vi "Enable-Disable.vi"(8 "error in (no error)":errorcluster, 10 "State":enum16{"Init", "Account Verified"}(ring), 11 "Control/Indicator References":T1) -> (0 "error out":errorcluster)   [LabVIEW 2020]
doc: "This VI enables/disables controls and indicators."
uses:
  Controls/Controls-Indicators References.ctl
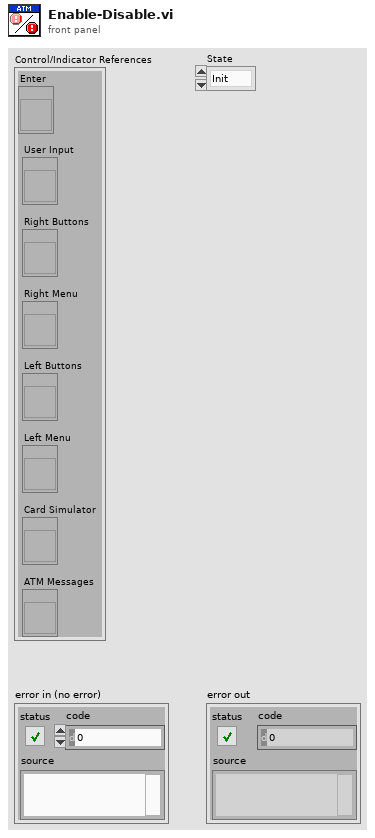
[diagram p1: front panel]
types:
  T1 = typedef "Controls-Indicators References.ctl" = cluster{"Enter":refnum<vi>, "User Input":refnum<vi>, "Right Buttons":refnum<vi>, "Right Menu":refnum<vi>, "Left Buttons":refnum<vi>, "Left Menu":refnum<vi>, "Card Simulator":refnum<vi>, "ATM Messages":refnum<vi>}
  T2 = enum8{"Enabled", "Disabled", "Disabled and Grayed Out"}
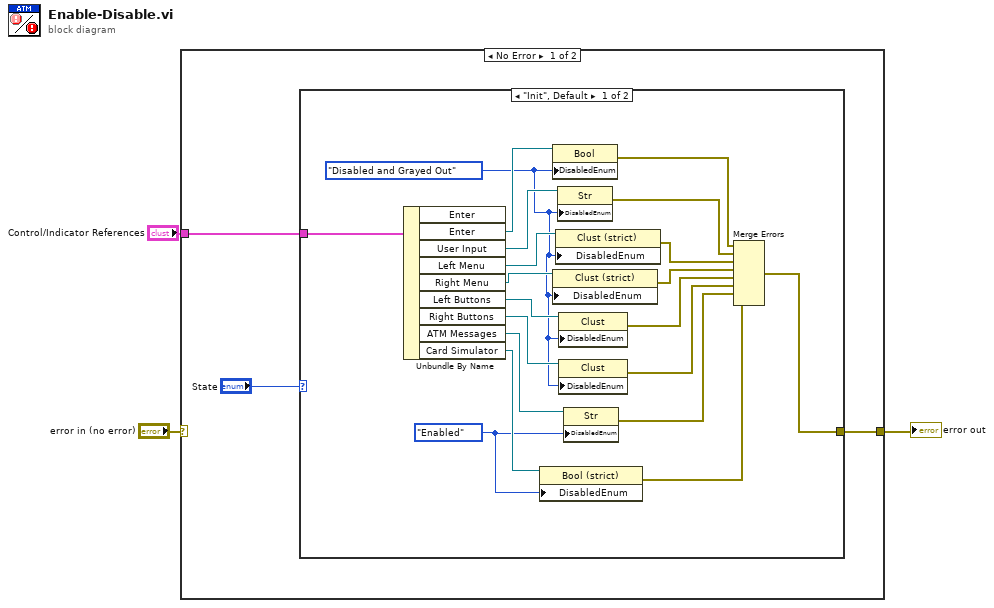
[diagram p0: block diagram]
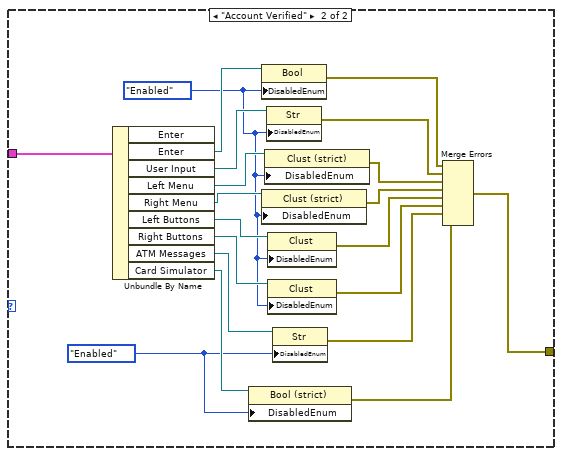
[diagram p2: hidden frame]
diagram:
  n1 = case shown="No Error" "error in (no error)" {
    selector: "error in (no error)" -> [_ w47]
    tunnel: [w5 w47] -> w2
    tunnel: "Control/Indicator References" -> [w6 _]
    frame No Error {
      n2 = case shown="\"Init\", Default" "State" {
        tunnel: w6 -> [w26 w46]
        tunnel: [w12 w32] -> w5
        frame "Init", Default {
          w7 = T2."Enabled" ("Disabled")
          w19 = T2."Disabled and Grayed Out" ("Disabled")
          n3 = Unbundle By Name(w26) -> ("Enter"=w25:refnum<vi>, "User Input"=w24:refnum<vi>, "Left Menu"=w23:refnum<vi>, "Right Menu"=w22:refnum<vi>, "Left Buttons"=w21:refnum<vi>, "Right Buttons"=w20:refnum<vi>, "ATM Messages"=w11:refnum<vi>, "Card Simulator"=w10:refnum<vi>)  [unwired: 1 out]
          n4 = property class="Bool (strict)"(reference=w10, "DisabledEnum"=w7) -> (error out=w8:errorcluster)  [unwired: 1 in, 1 out]
          n5 = property class="Bool"(reference=w25, "DisabledEnum"=w19) -> (error out=w18:errorcluster)  [unwired: 1 in, 1 out]
          n6 = property class="Clust (strict)"(reference=w22, "DisabledEnum"=w19) -> (error out=w15:errorcluster)  [unwired: 1 in, 1 out]
          n7 = property class="Clust (strict)"(reference=w23, "DisabledEnum"=w19) -> (error out=w16:errorcluster)  [unwired: 1 in, 1 out]
          n8 = property class="Str"(reference=w24, "DisabledEnum"=w19) -> (error out=w17:errorcluster)  [unwired: 1 in, 1 out]
          n9 = property class="Clust"(reference=w21, "DisabledEnum"=w19) -> (error out=w14:errorcluster)  [unwired: 1 in, 1 out]
          n10 = property class="Clust"(reference=w20, "DisabledEnum"=w19) -> (error out=w13:errorcluster)  [unwired: 1 in, 1 out]
          n11 = property class="Str"(reference=w11, "DisabledEnum"=w7) -> (error out=w9:errorcluster)  [unwired: 1 in, 1 out]
          n12 = Merge Errors(w18, w17, w16, w15, w14, w13, w9, w8) -> (w12:errorcluster)
        }
        frame "Account Verified" {
          w27 = T2."Enabled" ("Disabled")
          w39 = T2."Enabled" ("Disabled")
          n13 = Unbundle By Name(w46) -> ("Enter"=w45:refnum<vi>, "User Input"=w44:refnum<vi>, "Left Menu"=w43:refnum<vi>, "Right Menu"=w42:refnum<vi>, "Left Buttons"=w41:refnum<vi>, "Right Buttons"=w40:refnum<vi>, "ATM Messages"=w31:refnum<vi>, "Card Simulator"=w30:refnum<vi>)  [unwired: 1 out]
          n14 = property class="Bool (strict)"(reference=w30, "DisabledEnum"=w27) -> (error out=w28:errorcluster)  [unwired: 1 in, 1 out]
          n15 = property class="Bool"(reference=w45, "DisabledEnum"=w39) -> (error out=w38:errorcluster)  [unwired: 1 in, 1 out]
          n16 = property class="Clust (strict)"(reference=w42, "DisabledEnum"=w39) -> (error out=w35:errorcluster)  [unwired: 1 in, 1 out]
          n17 = property class="Clust (strict)"(reference=w43, "DisabledEnum"=w39) -> (error out=w36:errorcluster)  [unwired: 1 in, 1 out]
          n18 = property class="Str"(reference=w44, "DisabledEnum"=w39) -> (error out=w37:errorcluster)  [unwired: 1 in, 1 out]
          n19 = property class="Clust"(reference=w41, "DisabledEnum"=w39) -> (error out=w34:errorcluster)  [unwired: 1 in, 1 out]
          n20 = property class="Clust"(reference=w40, "DisabledEnum"=w39) -> (error out=w33:errorcluster)  [unwired: 1 in, 1 out]
          n21 = property class="Str"(reference=w31, "DisabledEnum"=w27) -> (error out=w29:errorcluster)  [unwired: 1 in, 1 out]
          n22 = Merge Errors(w38, w37, w36, w35, w34, w33, w29, w28) -> (w32:errorcluster)
        }
      }
    }
    frame Error {
    }
  }
  "error out" <- w2
